vi "Untitled 1 (SubVI).vi"(11 "VISAResourceName in":refnum<vi>) -> (0 "error out":errorcluster, 1 "error out 2":errorcluster, 2 "Speed 3":dbl, 3 "read buffer":string)   [LabVIEW 2016]
uses:
  <vilib>/Instr/_visa.llb/VISA Configure Serial Port (Instr).vi
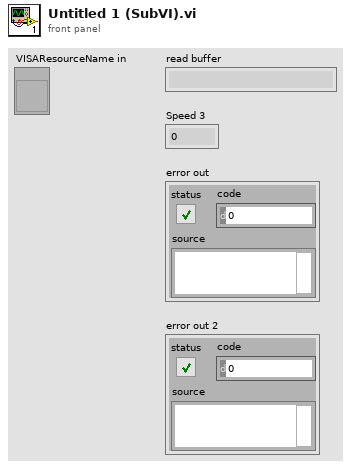
[diagram p1: front panel]
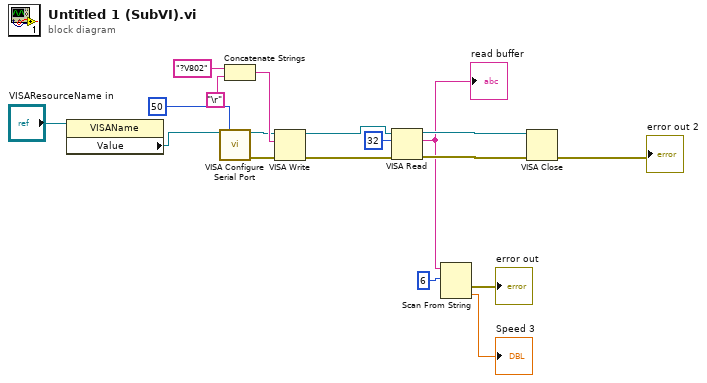
[diagram p0: block diagram]
diagram:
  n1 = property class="VISAName"(reference="VISAResourceName in") -> ("Value"=w5:refnum<visa-resource-name>)  [unwired: 1 in, 2 out]
  n2 = call-poly "VISA Configure Serial Port"("VISA resource name"=w5, "timeout (10sec)"=u32 50) -> ("VISA resource name out"=w16:refnum<visa-resource-name>, "error out"=w15:errorcluster)  [unwired: 12 in]
  n3 = Concatenate Strings("?V802" ("write buffer"), "\r") -> (w17:string)
  n4 = VISA Write(VISA resource name=w16, write buffer=w17, error in (no error)=w15) -> (VISA resource name out=w3:refnum<visa-resource-name>, error out=w2:errorcluster)  [unwired: 1 out]
  n5 = VISA Read(VISA resource name=w3, byte count=u32 32, error in (no error)=w2) -> (VISA resource name out=w12:refnum<visa-resource-name>, read buffer=w6:string, error out=w13:errorcluster)  [unwired: 1 out]
  "read buffer" <- w6
  n6 = Scan From String(input string=w6, initial scan location=u32 6) -> (error out=→"error out":errorcluster, output 1=→"Speed 3":dbl)  [unwired: 3 in, 2 out]
  n7 = VISA Close(VISA resource name=w12, error in (no error)=w13) -> (error out=→"error out 2":errorcluster)
